vi "All Itegration Tests.vi"(8 "error in (no error)":errorcluster) -> (0 "error out":errorcluster)   [LabVIEW 2026, in "Tests.lvlib"]
doc: "Aggregator for the Lumberjack unit tier. Holds every pure-VI unit test as a parallel subVI so the whole tier runs from one call. Has no assertions itself; each child registers its own via Define Test. Run directly for a fast, fixture-free unit-only pass (interactive Caraya dialog), or let Test.vi call it inside the suite for a headless, reported run. Add a unit test by dropping it here in parallel (Test-Strategy 3.2, 6)."
uses:
  Tests.lvlib
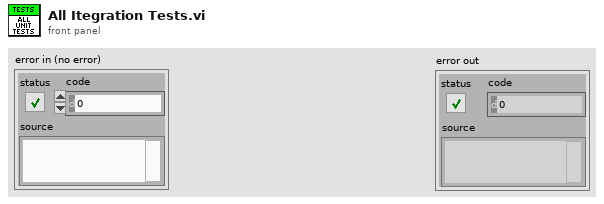
[diagram p1: front panel]
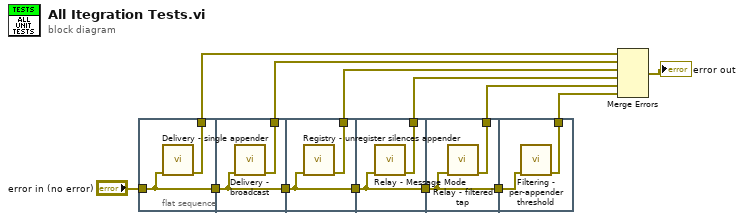
[diagram p0: block diagram]
diagram:
  n1 = flat-sequence {
    tunnel: "error in (no error)" -> [w14]
    tunnel: [w15] -> w9
    tunnel: [w14] -> w12
    tunnel: [w16] -> w13
    tunnel: w12 -> [w16]
    tunnel: [w17] -> w8
    tunnel: w13 -> [w18]
    tunnel: [w19] -> w7
    tunnel: [w18] -> w11
    tunnel: w11 -> [w20]
    tunnel: [w21] -> w6
    tunnel: [w20] -> w10
    tunnel: w10 -> [w22]
    tunnel: [w23] -> w5
    tunnel: [w22] -> w2
    tunnel: w2 -> [w25]
    tunnel: [w24] -> w1
    frame #0 {
      n2 = call "Delivery - single appender.vi"("error in (no error)"=w14) -> ("error out"=w15:errorcluster)  [unwired: 10 in]
    }
    frame #1 {
      n3 = call "Delivery - broadcast.vi"("error in (no error)"=w16) -> ("error out"=w17:errorcluster)  [unwired: 10 in]
    }
    frame #2 {
      n4 = call "Registry - unregister silences appender.vi"("error in (no error)"=w18) -> ("error out"=w19:errorcluster)  [unwired: 10 in]
    }
    frame #3 {
      n5 = call "Relay - Message Mode.vi"("error in (no error)"=w20) -> ("error out"=w21:errorcluster)  [unwired: 10 in]
    }
    frame #4 {
      n6 = call "Relay - filtered tap.vi"("error in (no error)"=w22) -> ("error out"=w23:errorcluster)  [unwired: 10 in]
    }
    frame #5 {
      n7 = call "Filtering - per-appender threshold.vi"("error in (no error)"=w25) -> ("error out"=w24:errorcluster)  [unwired: 10 in]
    }
  }
  n8 = Merge Errors(w9, w8, w7, w6, w5, w1) -> (→"error out":errorcluster)
